vi "MKS_PDR2000_read_unit.vi"(0 "PDR2000 COM port":refnum<visa-resource-name>, 11 "error in (no error)":errorcluster) -> (4 "PDR2000 COM port out":refnum<visa-resource-name>, 13 "Unit":string, 15 "error out":errorcluster)   [LabVIEW 2019]
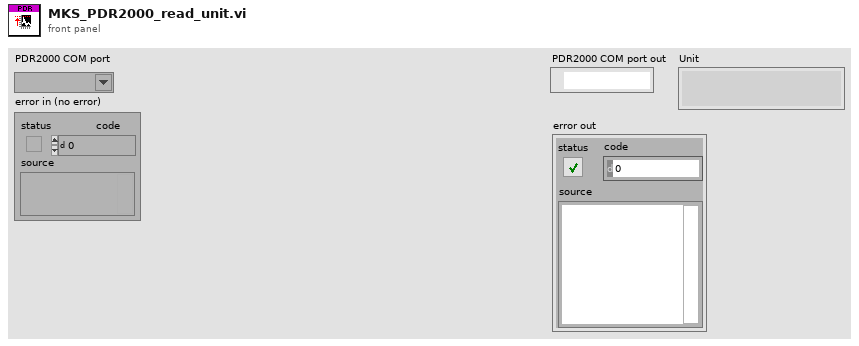
[diagram p1: front panel]
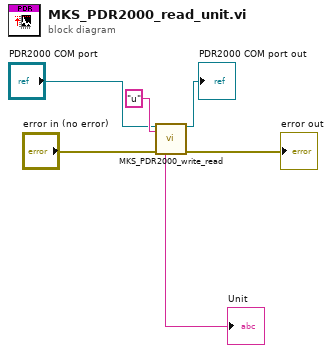
[diagram p0: block diagram]
diagram:
  n1 = call "MKS_PDR2000_write_read.vi"("PDR2000 COM port"="PDR2000 COM port", "Write string"="u", "error in (no error)"="error in (no error)") -> ("PDR2000 COM port out"=→"PDR2000 COM port out":refnum<visa-resource-name>, "Read String"=→"Unit":string, "error out"=→"error out":errorcluster)  [unwired: 10 in]
